vi "Logger.File.Read.Serials.vi"(8 "error in":errorcluster, 10 "Properties":T1, 11 "file ref in":refnum<k34>) -> (0 "error out":errorcluster, 2 "Data":T5[](array[typedef]), 3 "file ref out":refnum<k34>)   [LabVIEW 2016]
uses:
  Logger.File.Serials.ctl
  Sequence/Sequence.Step.Status.ctl
  Logger.File.Properties.ctl
  Sequence/Sequence.Code.SerialFormat.ctl
  Sequence/Sequence.Counters.ctl
panel:
  in  "Status":T4
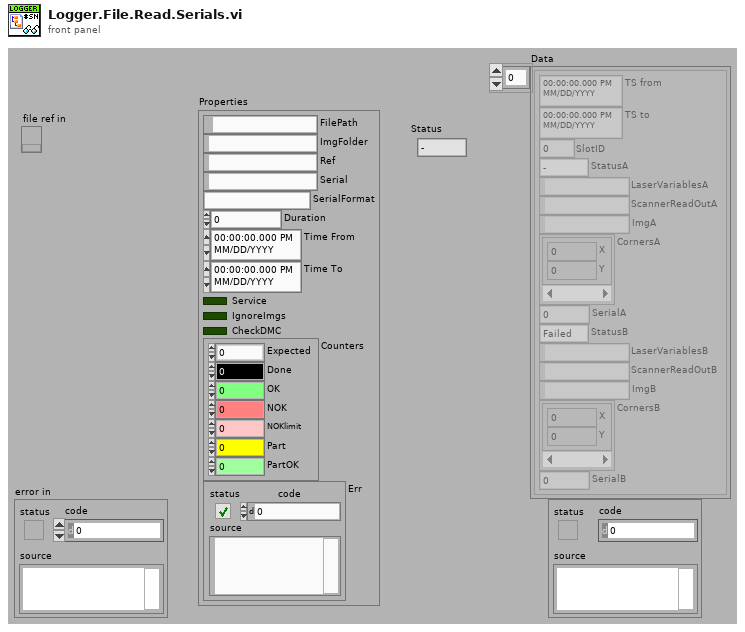
[diagram p1: front panel]
types:
  T1 = typedef "Logger.File.Properties.ctl" = cluster{"FilePath":path, "ImgFolder":string, "Ref":string, "Serial":string, "SerialFormat":T2, "Duration":dbl, "Time From":timestamp, "Time To":timestamp, "Service":bool, "IgnoreImgs":bool, "CheckDMC":bool, "Counters":T3, "Err":errorcluster}
  T2 = typedef "Sequence.Code.SerialFormat.ctl" = enum8{"", "6 dig", "7 dig"}
  T3 = typedef "Sequence.Counters.ctl" = cluster{"Expected":u16, "Done":u16, "OK":u16, "NOK":u16, "NOKlimit":u16, "Part":u16, "PartOK":u16}
  T4 = typedef "Sequence.Step.Status.ctl" = enum16{"-", "Pending", "Running", "Skipped", "Passed", "Failed", "Done", "Error", "Aborted", "Stopped"}
  T5 = typedef "Logger.File.Serials.ctl" = cluster{"TS from":timestamp, "TS to":timestamp, "SlotID":u8, "StatusA":T4, "LaserVariablesA":string, "ScannerReadOutA":string, "ImgA":string, "CornersA":cluster{"X":i32, "Y":i32}[], "SerialA":u8, "StatusB":T4, "LaserVariablesB":string, "ScannerReadOutB":string, "ImgB":string, "CornersB":cluster{"X":i32, "Y":i32}[], "SerialB":u8}
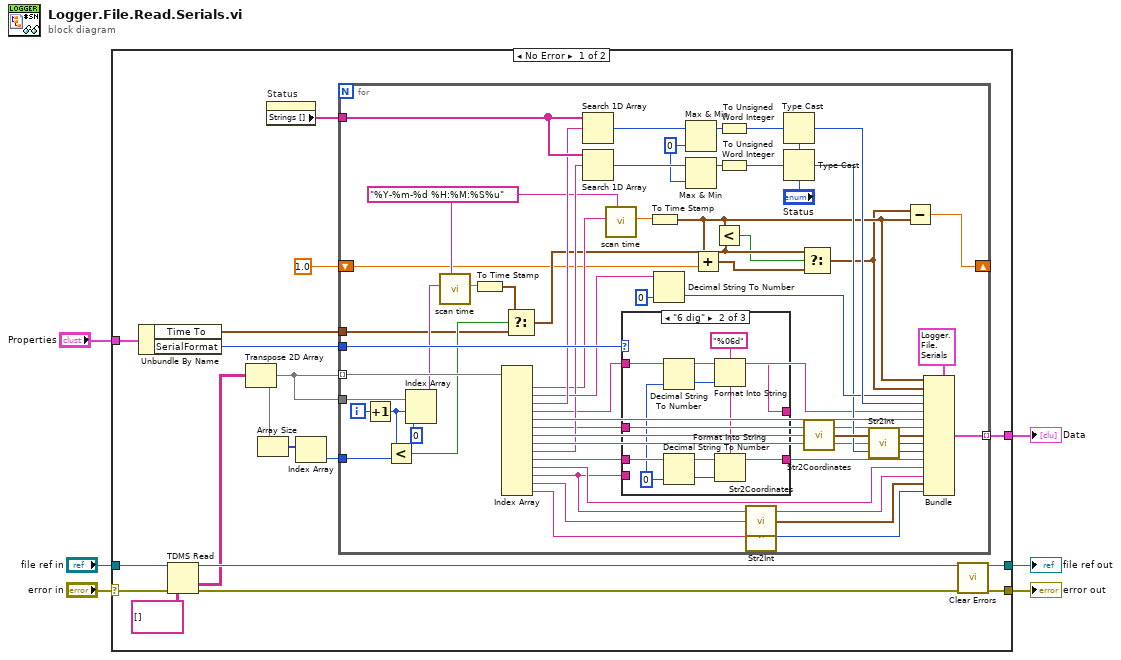
[diagram p0: block diagram]
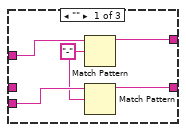
[diagram p2: hidden frame]
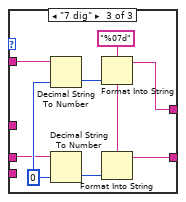
[diagram p3: hidden frame]
diagram:
  n1 = case shown="No Error" "error in" {
    selector: "error in" -> [w20 w99]
    tunnel: [w19 w99] -> w6
    tunnel: "file ref in" -> [w21 w98]
    tunnel: [w16 w98] -> w5
    tunnel: [w18 _] -> w2
    tunnel: "Properties" -> [w13 _]
    frame No Error {
      n2 = Unbundle By Name(w13) -> ("Time To"=w11:timestamp, "SerialFormat"=w12:T2)
      n3 = TDMS Read(0:w21, 11:w20, 12:string[][] [] ("appended array")) -> (4:w16:refnum<k34>, 10:w15:string[][], 15:w22:errorcluster)  [unwired: 5 in, 3 out]
      n4 = Transpose 2D Array(2D array=w15) -> (transposed array=w10:string[][])
      n5 = Array Size(array=w10) -> (size(s)=w9:i32[])
      n6 = property on="Status" class="Enum (strict)"() -> ("Strings []"=w14:string[])  [unwired: 2 in, 2 out]
      n7 = Index Array(array=w9) -> (element=w8:i32)  [unwired: 1 in]
      n8 = for {
        tunnel: w10 -> [w73] mode=indexing
        tunnel: [w76] -> w18 mode=indexing
        tunnel: w14 -> [w75]
        tunnel: w12 -> [w74]
        tunnel: w10 -> [w72]
        tunnel: w11 -> [w33]
        tunnel: w8 -> [w36]
        shift-right: [w32] -> _
        shift-left: 1.0 -> [w29]
        i -> [w71]
        w39 = "%Y-%m-%d %H:%M:%S%u" ("time format string")
        w25 = 0 ("y")
        n9 = Increment(x=w71) -> (x+1=w37:i32)
        n10 = Less?(x=w37, y=w36) -> (x < y?=w35:bool)
        n11 = Index Array(array=w72, index (row)=w37, index (col)=0 ("disabled index (col)")) -> (element=w40:string)
        n12 = call "scan time.vi"("time format string"=w39, "formatted time string"=w40) -> ("lv time (UTC)"=w42:dbl)  [unwired: 5 in, 4 out]
        n13 = To Time Stamp(1:w42) -> (0:w34:timestamp)
        n14 = Index Array(array=w73) -> (element #1=w38:string, element #2=w60:string, element #3=w66:string, element #4=w24:string, element #5=w58:string, element #6=w43:string, element #7=w56:string, element #8=w47:string, element #9=w46:string, element #10=w23:string, element #11=w52:string, element #12=w44:string, element #13=w50:string, element #14=w49:string)  [unwired: 14 in]
        n15 = Select(t=w34, s=w35, f=w33) -> (s? t:f=w31:timestamp)
        n16 = Search 1D Array(1D array=w75, element=w66) -> (index of element=w69:i32)  [unwired: 1 in]
        n17 = Search 1D Array(1D array=w75, element=w46) -> (index of element=w63:i32)  [unwired: 1 in]
        n18 = call "scan time.vi"("time format string"=w39, "formatted time string"=w38) -> ("lv time (UTC)"=w45:dbl)  [unwired: 5 in, 4 out]
        n19 = case shown="\"6 dig\"" w74 {
          tunnel: w24 -> [_ w88 w96]
          tunnel: [w78 w83 w91] -> _
          tunnel: [w80 w82 w90] -> _
          tunnel: w23 -> [_ w87 w95]
          tunnel: w44 -> [w81 _ _]
          tunnel: w43 -> [w79 _ _]
          frame "" {
            w77 = "-" ("regular expression")
            n20 = Match Pattern(string=w79, regular expression=w77) -> (before substring=w78:string)  [unwired: 1 in, 3 out]
            n21 = Match Pattern(string=w81, regular expression=w77) -> (before substring=w80:string)  [unwired: 1 in, 3 out]
          }
          frame "6 dig" {
            w84 = "%06d" ("format string")
            w89 = u32 0 ("default (0 I32)")
            n22 = Decimal String To Number(string=w88, default (0L)=w89) -> (number=w86:u32)  [unwired: 1 in, 1 out]
            n23 = Decimal String To Number(string=w87, default (0L)=w89) -> (number=w85:u32)  [unwired: 1 in, 1 out]
            n24 = Format Into String(format string=w84, w86) -> (resulting string=w83:string)  [unwired: 2 in, 1 out]
            n25 = Format Into String(format string=w84, w85) -> (resulting string=w82:string)  [unwired: 2 in, 1 out]
          }
          frame "7 dig" {
            w92 = "%07d" ("format string")
            w97 = u32 0 ("default (0 I32)")
            n26 = Decimal String To Number(string=w96, default (0L)=w97) -> (number=w94:u32)  [unwired: 1 in, 1 out]
            n27 = Decimal String To Number(string=w95, default (0L)=w97) -> (number=w93:u32)  [unwired: 1 in, 1 out]
            n28 = Format Into String(format string=w92, w94) -> (resulting string=w91:string)  [unwired: 2 in, 1 out]
            n29 = Format Into String(format string=w92, w93) -> (resulting string=w90:string)  [unwired: 2 in, 1 out]
          }
        }
        n30 = To Time Stamp(1:w45) -> (0:w30:timestamp)
        n31 = Decimal String To Number(string=w60, default (0L)=u8 0 ("default (0 I32)")) -> (number=w57:u8)  [unwired: 1 in, 1 out]
        n32 = Max & Min(x=w69, y=w25) -> (max(x,y)=w68:i32)  [unwired: 1 out]
        n33 = Max & Min(x=w63, y=w25) -> (max(x,y)=w64:i32)  [unwired: 1 out]
        n34 = Add(x=w30, y=w29) -> (x+y=w27:timestamp)
        n35 = Less?(x=w30, y=w31) -> (x < y?=w28:bool)
        n36 = To Unsigned Word Integer(number=w68) -> (unsigned 16bit integer=w67:u16)
        n37 = To Unsigned Word Integer(number=w64) -> (unsigned 16bit integer=w65:u16)
        n38 = call "Str2Coordinates.vi"("String"=w50) -> ("Coordinates"=w51:cluster{"X":dbl, "Y":dbl}[])  [unwired: 1 in]
        n39 = call "Str2Int.vi"("string"=w49) -> ("Numeric"=w48:i32)
        n40 = Type Cast(type="Status", x=w67) -> (*(type *) &x=w61:T4)
        n41 = Type Cast(type="Status", x=w65) -> (*(type *) &x=w54:T4)
        n42 = Select(t=w31, s=w28, f=w27) -> (s? t:f=w26:timestamp)
        n43 = call "Str2Coordinates.vi"("String"=w56) -> ("Coordinates"=w55:cluster{"X":dbl, "Y":dbl}[])  [unwired: 1 in]
        n44 = call "Str2Int.vi"("string"=w47) -> ("Numeric"=w53:i32)
        n45 = Subtract(x=w26, y=w30) -> (x-y=w32:dbl)
        n46 = Bundle(cluster=T5 {"TS from"=timestamp(0 s since 1904-01-01), "TS to"=timestamp(0 s since 1904-01-01), "SlotID"=0, "StatusA"=enum."-", "LaserVariablesA"="", "ScannerReadOutA"="", "ImgA"="", "CornersA"=[], "SerialA"=0, "StatusB"=enum."Failed", "LaserVariablesB"="", "ScannerReadOutB"="", "ImgB"="", "CornersB"=[], "SerialB"=0} ("SerialData"), "TS from"=w30, "TS to"=w26, "SlotID"=w57, "StatusA"=w61, "LaserVariablesA"=w24, "ScannerReadOutA"=w58, "ImgA"=w43, "CornersA"=w55, "SerialA"=w53, "StatusB"=w54, "LaserVariablesB"=w23, "ScannerReadOutB"=w52, "ImgB"=w44, "CornersB"=w51, "SerialB"=w48) -> (w76:T5)
      }
      n47 = call <vilib>:"Clear Errors.vi"("error in (no error)"=w22) -> ("error out"=w19:errorcluster)  [unwired: 5 in, 1 out]
    }
    frame Error {
    }
  }
  "error out" <- w6
  "file ref out" <- w5
  "Data" <- w2
